vi "Exchange Table array.vi"(5 "Exchange Table":T1) -> (2 "appended array":string[](array[string]))   [LabVIEW 2014]
uses:
  Type'def/Exchange Table.ctl
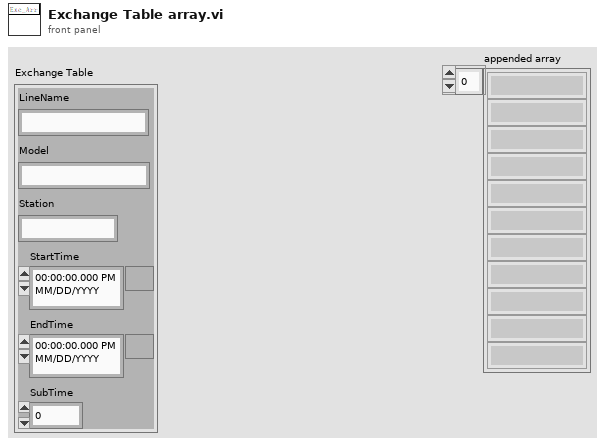
[diagram p1: front panel]
types:
  T1 = typedef "Exchange Table.ctl" = cluster{"LineName":string, "Model":string, "Station":string, "StartTime":timestamp, "EndTime":timestamp, "SubTime":dbl}
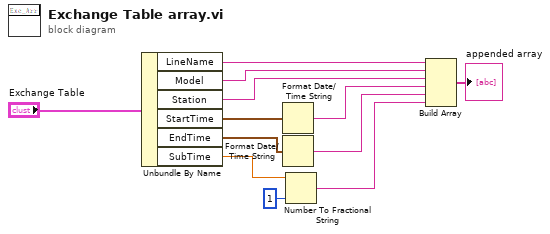
[diagram p0: block diagram]
diagram:
  n1 = Unbundle By Name("Exchange Table") -> ("LineName"=w11:string, "Model"=w10:string, "Station"=w9:string, "StartTime"=w8:timestamp, "EndTime"=w6:timestamp, "SubTime"=w4:dbl)
  n2 = Format Date/Time String(seconds (now)=w8) -> (date/time string=w7:string)  [unwired: 2 in]
  n3 = Format Date/Time String(seconds (now)=w6) -> (date/time string=w5:string)  [unwired: 2 in]
  n4 = Number To Fractional String(number=w4, precision (6)=i16 1) -> (F-format string=w3:string)  [unwired: 2 in]
  n5 = Build Array(w11, w10, w9, w7, w5, w3) -> (→"appended array":string[])
